vi "Update PID data in MeasDataQ.vi"(4 "UpdateTS (T)":bool=TRUE, 7 "WeldGapMeas":T1, 8 "error in (no error)":errorcluster, 9 "TimeStamp":timestamp) -> (0 "error out":errorcluster, 3 "orData out":T2)   [LabVIEW 2017]
doc: "Developed by Kevin Thompson\nThompson Engineering, LLC\nkevin@thompsonengineering.net"
uses:
  TD MeasData QRef.ctl
  TD MeasData--cluster.ctl
  GBL DataQ Ref.vi
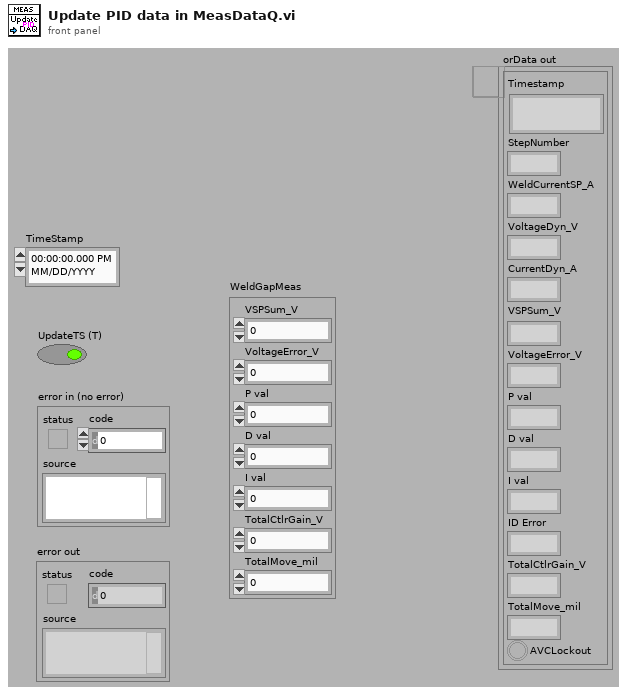
[diagram p1: front panel]
types:
  T1 = cluster{"VSPSum_V":dbl, "VoltageError_V":dbl, "P val":dbl, "D val":dbl, "I val":dbl, "TotalCtlrGain_V":dbl, "TotalMove_mil":dbl}
  T2 = typedef "TD MeasData QRef.ctl" = refnum<queue>
  T3 = typedef "TD MeasData--cluster.ctl" = cluster{"Timestamp":timestamp, "StepNumber":i32, "WeldCurrentSP_A":dbl, "VoltageDyn_V":dbl, "CurrentDyn_A":dbl, "VSPSum_V":dbl, "VoltageError_V":dbl, "P val":dbl, "D val":dbl, "I val":dbl, "ID Error":dbl, "TotalCtlrGain_V":dbl, "TotalMove_mil":dbl, "AVCLockout":bool}
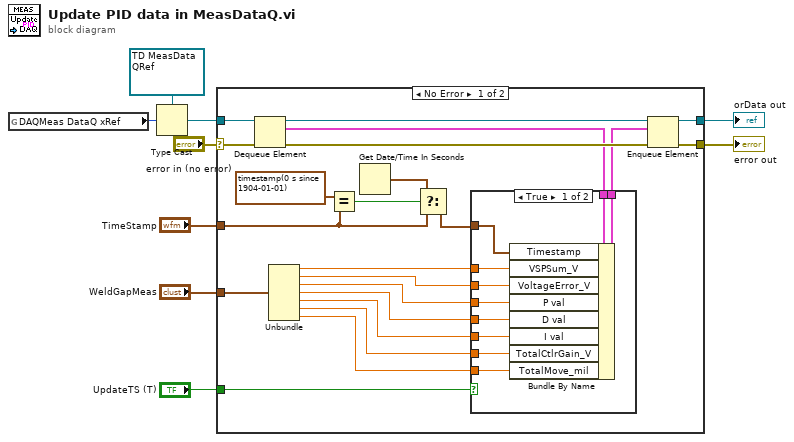
[diagram p0: block diagram]
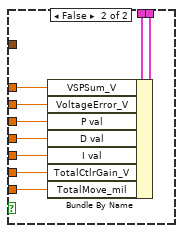
[diagram p2: hidden frame]
diagram:
  n1 = global read "GBL DataQ Ref.vi" "DAQMeas DataQ xRef"() -> (w3:u32)
  n2 = Type Cast(type=T2 refnum ("orData in"), x=w3) -> (*(type *) &x=w5:T2)
  n3 = case shown="No Error" "error in (no error)" {
    selector: "error in (no error)" -> [w26 w51]
    tunnel: w5 -> [w31 w52]
    tunnel: [w28 w51] -> w9
    tunnel: [w27 w52] -> w8
    tunnel: "TimeStamp" -> [w21 _]
    tunnel: "WeldGapMeas" -> [w18 _]
    tunnel: "UpdateTS (T)" -> [w10 _]
    frame No Error {
      n4 = Dequeue Element(queue=w31, error in (no error)=w26) -> (queue out=w29:T2, element=w25:T3, error out=w30:errorcluster)  [unwired: 1 in, 1 out]
      n5 = Unbundle(w18) -> ("VSPSum_V"=w17:dbl, "VoltageError_V"=w16:dbl, "P val"=w15:dbl, "D val"=w14:dbl, "I val"=w13:dbl, "TotalCtlrGain_V"=w12:dbl, "TotalMove_mil"=w11:dbl)
      n6 = Equal?(x=timestamp(0 s since 1904-01-01) ("TimeStamp"), y=w21) -> (x = y?=w22:bool)
      n7 = Get Date/Time In Seconds() -> (seconds since 1Jan1904=w19:timestamp)
      n8 = Select(t=w19, s=w22, f=w21) -> (s? t:f=w20:timestamp)
      n9 = case shown="True" w10 {
        tunnel: w25 -> [w41 w50]
        tunnel: [w40 w49] -> w24
        tunnel: w20 -> [w39 _]
        tunnel: w17 -> [w38 w48]
        tunnel: w16 -> [w37 w47]
        tunnel: w15 -> [w36 w46]
        tunnel: w14 -> [w35 w45]
        tunnel: w13 -> [w34 w44]
        tunnel: w12 -> [w33 w43]
        tunnel: w11 -> [w32 w42]
        frame True {
          n10 = Bundle By Name(cluster=w41, "Timestamp"=w39, "VSPSum_V"=w38, "VoltageError_V"=w37, "P val"=w36, "D val"=w35, "I val"=w34, "TotalCtlrGain_V"=w33, "TotalMove_mil"=w32) -> (w40:T3)
        }
        frame False {
          n11 = Bundle By Name(cluster=w50, "VSPSum_V"=w48, "VoltageError_V"=w47, "P val"=w46, "D val"=w45, "I val"=w44, "TotalCtlrGain_V"=w43, "TotalMove_mil"=w42) -> (w49:T3)
        }
      }
      n12 = Enqueue Element(queue=w29, element=w24, error in (no error)=w30) -> (queue out=w27:T2, error out=w28:errorcluster)  [unwired: 1 in, 1 out]
    }
    frame Error {
    }
  }
  "orData out" <- w8
  "error out" <- w9
